vi "Import_xy-wiArray.old.vi"(5 "InputArray":dbl[][](array[numeric]) format="%0.3f", 7 "Uniform":bool) -> (0 "XY Full":cluster{dbl, dbl}[](array[cluster]), 1 "XY Unique":cluster{"X Unique":dbl[], "Y Unique":dbl[]}, 2 "Wavelength":dbl[](array[numeric]), 3 "Intensity":dbl[][](array[numeric]), 4 "XY Full Interpol.":cluster{dbl, dbl}[](array[cluster]), 6 "Axes":T1)   [LabVIEW 2010]
uses:
  <vilib>/Analysis/polynomials.llb/Unique Numbers and Multiplicity (DBL).vi
  <vilib>/Analysis/NI_AALPro.lvlib
  <vilib>/Analysis/NI_AALBase.lvlib
panel:
  # "Imports a 2D-array containing XY-WI data. XY varies over columns, XY-data are stored in the first two rows, respctively.\nW (wavelength/Raman shift) varies over rows."
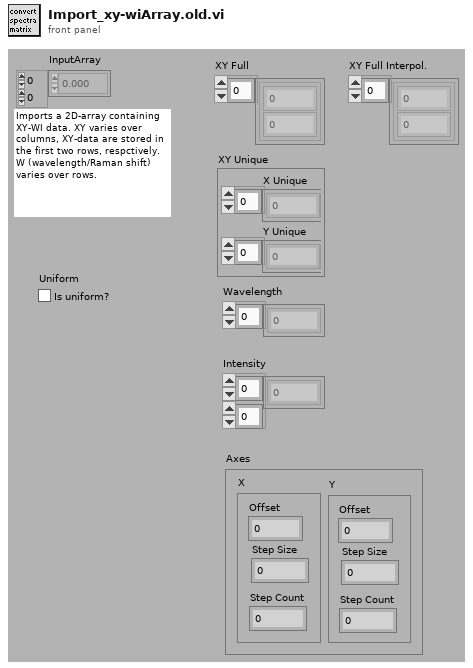
[diagram p1: front panel]
types:
  T1 = cluster{"X":cluster{"Offset":dbl, "Step Size":dbl, "Step Count":i32}, "Y":cluster{"Offset":dbl, "Step Size":dbl, "Step Count":i32}}
  T2 = cluster{"closest element":dbl, "closest element":dbl}[]
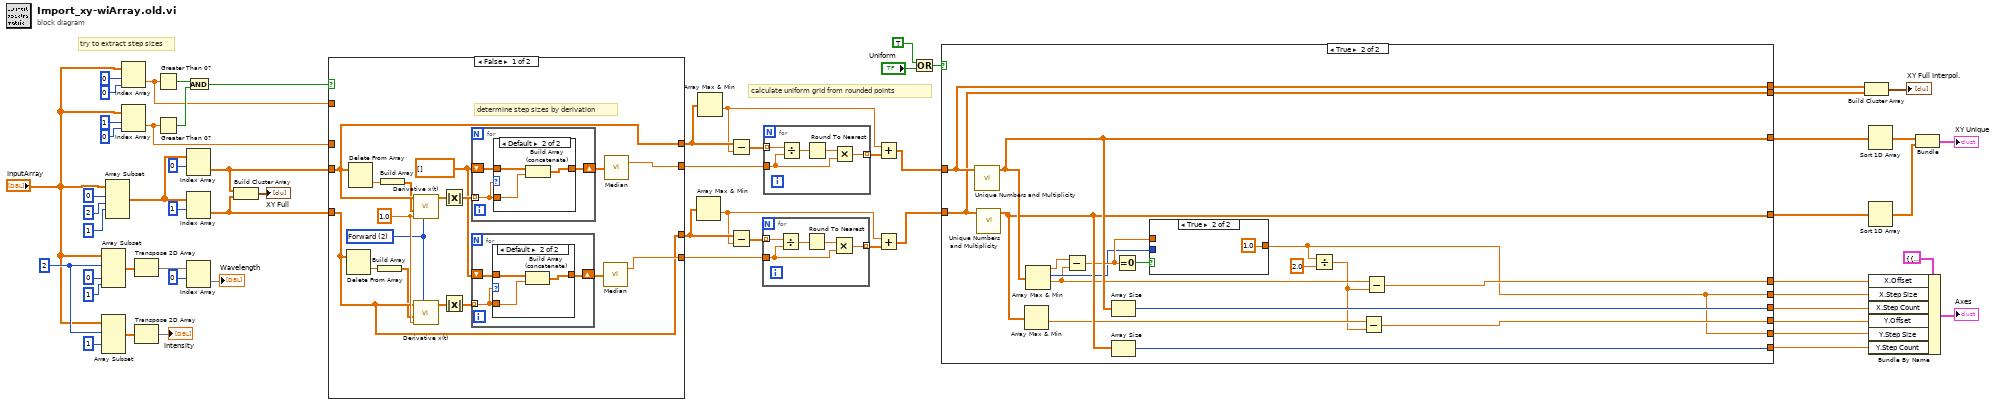
[diagram p0: block diagram]
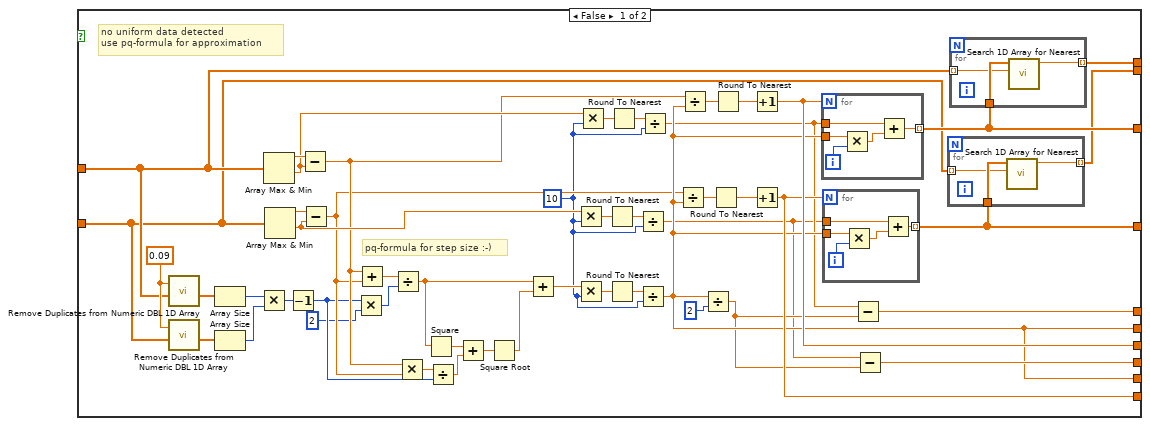
[diagram p5: hidden frame]
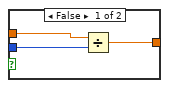
[diagram p6: hidden frame]
diagram:
  w56 = 2 ("Index")
  # "calculate uniform grid from rounded points"
  # "try to extract step sizes"
  n1 = Array Subset(array="InputArray", index (row)=w56, index (col)=0 ("Index"), length (col)=1 ("Länge")) -> (w53:dbl[][])  [unwired: 1 in]
  n2 = Array Subset(array="InputArray", index (row)=w56, index (col)=1 ("Index")) -> (w51:dbl[][])  [unwired: 2 in]
  n3 = Array Subset(array="InputArray", index (row)=0 ("Index"), length (row)=2 ("Länge"), index (col)=1 ("Index")) -> (w45:dbl[][])  [unwired: 1 in]
  n4 = Index Array(array="InputArray", index (row)=0, index (col)=0 ("disabled index (col)")) -> (element=w22:dbl)
  n5 = Index Array(array="InputArray", index (row)=1, index (col)=0 ("disabled index (col)")) -> (element=w21:dbl)
  n6 = Transpose 2D Array(2D array=w53) -> (transposed array=w52:dbl[][])
  n7 = Transpose 2D Array(2D array=w51) -> (transposed array=→"Intensity":dbl[][])
  n8 = Greater Than 0?(x=w22) -> (x > 0?=w26:bool)
  n9 = Greater Than 0?(x=w21) -> (x > 0?=w27:bool)
  n10 = Index Array(array=w45, index (row)=0 ("Index (Zeile)")) -> (element=w18:dbl[])  [unwired: 1 in]
  n11 = Index Array(array=w45, index (row)=1 ("Index (Zeile)")) -> (element=w17:dbl[])  [unwired: 1 in]
  n12 = Index Array(array=w52, index (row)=0 ("Index")) -> (element=→"Wavelength":dbl[])  [unwired: 1 in]
  n13 = And(x=w26, y=w27) -> (x .and. y?=w20:bool)
  n14 = Build Cluster Array(w18, w17) -> (→"XY Full":cluster{dbl, dbl}[])
  n15 = case shown="False" w20 {
    tunnel: w18 -> [w65 w93]
    tunnel: w17 -> [w66 w94]
    tunnel: w22 -> [_ w92]
    tunnel: w21 -> [_ w95]
    tunnel: [w67 w95] -> w13
    tunnel: [w66 w94] -> w5
    tunnel: [w65 w93] -> w10
    tunnel: [w68 w92] -> w12
    frame False {
      w71 = dbl[] [] ("abs(x)")
      w69 = u16 2 items=["2nd Order Central", "4th Order Central", "Forward", "Backward"] ("method")
      w70 = 1.0 ("dt")
      # "determine step sizes by derivation"
      n16 = Delete From Array(array=w66) -> (deleted portion=w64:dbl)  [unwired: 2 in, 1 out]
      n17 = Delete From Array(array=w65) -> (deleted portion=w62:dbl)  [unwired: 2 in, 1 out]
      n18 = Build Array(w64) -> (w63:dbl[])
      n19 = Build Array(w62) -> (w61:dbl[])
      n20 = call <vilib>:"Derivative x(t).vi"("method"=w69, "dt"=w70, "Final Condition"=w61, "X"=w65) -> ("dX/dt"=w75:dbl[])  [unwired: 6 in, 1 out]
      n21 = call <vilib>:"Derivative x(t).vi"("method"=w69, "dt"=w70, "Final Condition"=w63, "X"=w66) -> ("dX/dt"=w72:dbl[])  [unwired: 6 in, 1 out]
      n22 = Absolute Value(x=w75) -> (abs(x)=w76:dbl[])
      n23 = Absolute Value(x=w72) -> (abs(x)=w73:dbl[])
      n24 = for {
        shift-right: [w79] -> w74
        shift-left: w71 -> [w80]
        tunnel: w73 -> [w78] mode=indexing
        n25 = case shown="Default" w78 {
          tunnel: w80 -> [w81 w84]
          tunnel: [w81 w83] -> w79
          tunnel: w78 -> [_ w82]
          frame 0 {
          }
          frame Default {
            n26 = Build Array (concatenate)(w84, w82) -> (w83:dbl[])
          }
        }
      }
      n27 = for {
        shift-right: [w86] -> w77
        shift-left: w71 -> [w87]
        tunnel: w76 -> [w85] mode=indexing
        n28 = case shown="Default" w85 {
          tunnel: w87 -> [w88 w91]
          tunnel: [w88 w90] -> w86
          tunnel: w85 -> [_ w89]
          frame 0 {
          }
          frame Default {
            n29 = Build Array (concatenate)(w91, w89) -> (w90:dbl[])
          }
        }
      }
      n30 = call <vilib>:"Median.vi"("X"=w74) -> ("median"=w67:dbl)  [unwired: 1 out]
      n31 = call <vilib>:"Median.vi"("X"=w77) -> ("median"=w68:dbl)  [unwired: 1 out]
    }
    frame True {
      # "step sizes detected"
    }
  }
  n32 = Array Max & Min(array=w5) -> (min value=w2:dbl)  [unwired: 3 out]
  n33 = Array Max & Min(array=w10) -> (min value=w7:dbl)  [unwired: 3 out]
  n34 = Subtract(x=w10, y=w7) -> (x-y=w9:dbl[])
  n35 = Subtract(x=w5, y=w2) -> (x-y=w4:dbl[])
  n36 = for {
    tunnel: w4 -> [w99] mode=indexing
    tunnel: w13 -> [w97]
    tunnel: [w96] -> w3 mode=indexing
    n37 = Divide(x=w99, y=w97) -> (x/y=w100:dbl)
    n38 = Round To Nearest(number=w100) -> (nearest integer value=w98:dbl)
    n39 = Multiply(x=w98, y=w97) -> (x*y=w96:dbl)
  }
  n40 = for {
    tunnel: w9 -> [w104] mode=indexing
    tunnel: w12 -> [w102]
    tunnel: [w101] -> w8 mode=indexing
    n41 = Divide(x=w104, y=w102) -> (x/y=w105:dbl)
    n42 = Round To Nearest(number=w105) -> (nearest integer value=w103:dbl)
    n43 = Multiply(x=w103, y=w102) -> (x*y=w101:dbl)
  }
  n44 = Add(x=w7, y=w8) -> (x+y=w6:dbl[])
  n45 = Add(x=w2, y=w3) -> (x+y=w1:dbl[])
  n46 = Or(x=TRUE, y="Uniform") -> (x .or. y?=w23:bool)
  n47 = case shown="True" w23 {
    tunnel: [w108 w185] -> w41
    tunnel: [w110 w187] -> w40
    tunnel: [w154 w186] -> w37
    tunnel: [w153 w184] -> w36
    tunnel: [w150 w173] -> w35
    tunnel: [w152 w174] -> w34
    tunnel: [w151 w175] -> w33
    tunnel: w6 -> [w111 w172]
    tunnel: w1 -> [w107 w171]
    tunnel: [w150 w173] -> w25
    tunnel: [w109 w172] -> w16
    tunnel: [w106 w171] -> w15
    frame False {
      w117 = 0.09 ("Tolerance (1E-9)")
      w124 = i8 10 ("y")
      # "no uniform data detected\nuse pq-formula for approximation"
      # "pq-formula for step size :-)"
      n48 = call "Remove Duplicates from Numeric DBL 1D Array.vi"("Tolerance (1E-9)"=w117, "Array In"=w111) -> ("Sorted Array with Duplicates Removed"=w112:dbl[])  [unwired: 8 in, 1 out]
      n49 = call "Remove Duplicates from Numeric DBL 1D Array.vi"("Tolerance (1E-9)"=w117, "Array In"=w107) -> ("Sorted Array with Duplicates Removed"=w113:dbl[])  [unwired: 8 in, 1 out]
      n50 = Array Size(array=w112) -> (size(s)=w115:i32)
      n51 = Array Size(array=w113) -> (size(s)=w116:i32)
      n52 = Multiply(x=w115, y=w116) -> (x*y=w114:i32)
      n53 = Array Max & Min(array=w111) -> (max value=w148:dbl, min value=w140:dbl)  [unwired: 2 out]
      n54 = Array Max & Min(array=w107) -> (max value=w149:dbl, min value=w145:dbl)  [unwired: 2 out]
      n55 = Decrement(x=w114) -> (x-1=w130:i32)
      n56 = Subtract(x=w148, y=w140) -> (x-y=w139:dbl)
      n57 = Subtract(x=w149, y=w145) -> (x-y=w138:dbl)
      n58 = Multiply(x=w130, y=2) -> (x*y=w136:i32)
      n59 = Add(x=w139, y=w138) -> (x+y=w137:dbl)
      n60 = Divide(x=w137, y=w136) -> (x/y=w133:dbl)
      n61 = Multiply(x=w139, y=w138) -> (x*y=w131:dbl)
      n62 = Square(x=w133) -> (x^2=w132:dbl)
      n63 = Divide(x=w131, y=w130) -> (x/y=w128:dbl)
      n64 = Add(x=w132, y=w128) -> (x+y=w134:dbl)
      n65 = Square Root(x=w134) -> (sqrt(x)=w135:dbl)
      n66 = Add(x=w133, y=w135) -> (x+y=w125:dbl)
      n67 = Multiply(x=w145, y=w124) -> (x*y=w144:dbl)
      n68 = Multiply(x=w125, y=w124) -> (x*y=w122:dbl)
      n69 = Multiply(x=w140, y=w124) -> (x*y=w142:dbl)
      n70 = Round To Nearest(number=w144) -> (nearest integer value=w143:dbl)
      n71 = Round To Nearest(number=w122) -> (nearest integer value=w123:dbl)
      n72 = Round To Nearest(number=w142) -> (nearest integer value=w141:dbl)
      n73 = Divide(x=w143, y=w124) -> (x/y=w118:dbl)
      n74 = Divide(x=w123, y=w124) -> (x/y=w150:dbl)
      n75 = Divide(x=w141, y=w124) -> (x/y=w119:dbl)
      n76 = Divide(x=w138, y=w150) -> (x/y=w146:dbl)
      n77 = Divide(x=w139, y=w150) -> (x/y=w147:dbl)
      n78 = Divide(x=w150, y=i8 2) -> (x/y=w120:dbl)
      n79 = Round To Nearest(number=w146) -> (nearest integer value=w126:dbl)
      n80 = Round To Nearest(number=w147) -> (nearest integer value=w127:dbl)
      n81 = Increment(x=w127) -> (x+1=w154:dbl)
      n82 = Increment(x=w126) -> (x+1=w153:dbl)
      n83 = for {
        N: w154 -> [_]
        tunnel: w119 -> [w164]
        tunnel: w150 -> [w162]
        tunnel: [w161] -> w110 mode=indexing
        i -> [w163]
        n84 = Multiply(x=w162, y=w163) -> (x*y=w165:dbl)
        n85 = Add(x=w164, y=w165) -> (x+y=w161:dbl)
      }
      n86 = for {
        N: w153 -> [_]
        tunnel: w118 -> [w169]
        tunnel: w150 -> [w167]
        tunnel: [w166] -> w108 mode=indexing
        i -> [w168]
        n87 = Multiply(x=w167, y=w168) -> (x*y=w170:dbl)
        n88 = Add(x=w169, y=w170) -> (x+y=w166:dbl)
      }
      n89 = Subtract(x=w119, y=w120) -> (x-y=w151:dbl)
      n90 = Subtract(x=w118, y=w120) -> (x-y=w152:dbl)
      n91 = for {
        tunnel: w107 -> [w156] mode=indexing
        tunnel: w108 -> [w157]
        tunnel: [w155] -> w106 mode=indexing
        n92 = call "Search 1D Array for Nearest.vi"("desired element"=w156, "1D Array"=w157) -> ("closest element"=w155:dbl)  [unwired: 8 in, 1 out]
      }
      n93 = for {
        tunnel: w111 -> [w159] mode=indexing
        tunnel: w110 -> [w160]
        tunnel: [w158] -> w109 mode=indexing
        n94 = call "Search 1D Array for Nearest.vi"("desired element"=w159, "1D Array"=w160) -> ("closest element"=w158:dbl)  [unwired: 8 in, 1 out]
      }
    }
    frame True {
      n95 = call-poly <vilib>:"Unique Numbers and Multiplicity.vi"("Numbers"=w172) -> ("Unique Numbers"=w187:dbl[])  [unwired: 8 in, 2 out]
      n96 = call-poly <vilib>:"Unique Numbers and Multiplicity.vi"("Numbers"=w171) -> ("Unique Numbers"=w185:dbl[])  [unwired: 8 in, 2 out]
      n97 = Array Max & Min(array=w185) -> (min value=w177:dbl)  [unwired: 3 out]
      n98 = Array Max & Min(array=w187) -> (max value=w183:dbl, max index (indices)=w180:i32, min value=w178:dbl)  [unwired: 1 out]
      n99 = Subtract(x=w183, y=w178) -> (x-y=w181:dbl)
      n100 = Array Size(array=w187) -> (size(s)=w186:i32)
      n101 = Array Size(array=w185) -> (size(s)=w184:i32)
      n102 = Equal To 0?(x=w181) -> (x = 0?=w182:bool)
      n103 = case shown="True" w182 {
        tunnel: w181 -> [w190 _]
        tunnel: w180 -> [w188 _]
        tunnel: [w189 1.0] -> w173
        frame False {
          n104 = Divide(x=w190, y=w188) -> (x/y=w189:dbl)
        }
        frame True {
        }
      }
      n105 = Divide(x=w173, y=2.0) -> (x/y=w176:dbl)
      n106 = Subtract(x=w177, y=w176) -> (x-y=w174:dbl)
      n107 = Subtract(x=w178, y=w176) -> (x-y=w175:dbl)
    }
  }
  n108 = Build Cluster Array(w16, w15) -> (→"XY Full Interpol.":T2)
  n109 = Sort 1D Array(array=w40) -> (sorted array=w43:dbl[])
  n110 = Sort 1D Array(array=w41) -> (sorted array=w42:dbl[])
  n111 = Bundle By Name(cluster=T1 {"X"={"Offset"=0.0, "Step Size"=0.0, "Step Count"=0}, "Y"={"Offset"=0.0, "Step Size"=0.0, "Step Count"=0}} ("Axes"), "X.Offset"=w33, "X.Step Size"=w35, "X.Step Count"=w37, "Y.Offset"=w34, "Y.Step Size"=w25, "Y.Step Count"=w36) -> (→"Axes":T1)
  n112 = Bundle(w43, w42) -> (→"XY Unique":cluster{dbl[], dbl[]})  [unwired: 1 in]
